vi "Set Com Address.vi"(10 "Com Address":u8, 11 "Tovey9150 in":refnum<class "Tovey 9150.lvclass">) -> (3 "Tovey9150 out":refnum<class "Tovey 9150.lvclass">)   [LabVIEW 2015, in "Tovey 9150.lvclass"]
uses:
  Tovey 9150.lvclass
  Tovey 9150.lvclass/Tovey 9150.ctl
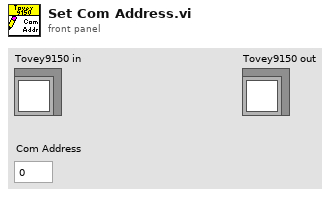
[diagram p1: front panel]
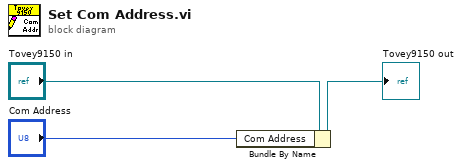
[diagram p0: block diagram]
diagram:
  n1 = Bundle By Name(cluster="Tovey9150 in", "Com Address"="Com Address") -> (→"Tovey9150 out":refnum<class "Tovey 9150.lvclass">)
